vi "main_ctrl.vi"(8 "error in":errorcluster) -> (0 "error out":errorcluster caption="error")   [LabVIEW 2013]
uses:
  <vilib>/Rock Robotics/WPI/DriverStation/WPI_DriverStationRobotMode.ctl
  typedefs/fg_typedef.ctl
  typedefs/vision enable.ctl
  typedefs/subStates.ctl
  typedefs/singleUseSubstate.ctl
  <vilib>/Rock Robotics/WPI/Solenoid/WPI_SolenoidValue.ctl
  <vilib>/Rock Robotics/WPI/Compressor/WPI_CompressorGetSetRefNum.vi
  <vilib>/Rock Robotics/WPI/RobotDrive/WPI_RobotDriveGetSetRefNum.vi
  <vilib>/Rock Robotics/WPI/RobotDrive/WPI_RobotDriveArcadeDrive_Standard(NoSaturation).vi
  <vilib>/Rock Robotics/WPI/Solenoid/WPI_SolenoidSetEnum.vi
panel:
  out "Robot Mode":T1
  out "Vision SPI":u32
  out "Vision IPS":dbl
  out "Main IPS":dbl
  out "Main SPI":u32
  # "MAIN CONTROL"
  # "holds robot control code - dual parallel state machine"
  # "SPI: milliseconds per iteration\nIPS: iterations per second"
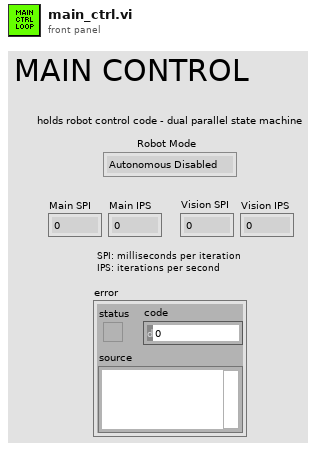
[diagram p1: front panel]
types:
  T1 = typedef "WPI_DriverStationRobotMode.ctl" = enum16{"Autonomous Disabled", "Autonomous Enabled", "Teleop Disabled", "Teleop Enabled", "Timeout", "Finish"}
  T2 = typedef "WPI_RobotDriveDevRef.ctl" = cluster{"DevStatus":errorcluster, "Motors[]":T3[], "Square Inputs":bool, "Max Output":dbl, "Isochronous":bool}
  T3 = typedef "WPI_MotorControlDeviceRef.ctl" = cluster{"DeviceStatus":errorcluster, "Type":enum16{"PWM", "CAN"}, "PWM":cluster{"Digital Module":T4, "PWM Channel":T5, "DeadBand":T6}, "CAN":cluster{"Device Number":u8, "Control Mode":T7, "Semaphore":T8, "Max Vout":dbl}, "Invert":bool, "TransformRef":T9, "InvTransformRef":T9}
  T4 = typedef "FPGA_TypedefDigitalModule.ctl" = enum16{"Digital Module 1", "Digital Module 2"}
  T5 = typedef "FPGA_DIOPWMChannel.ctl" = enum8{"PWM 1", "PWM 2", "PWM 3", "PWM 4", "PWM 5", "PWM 6", "PWM 7", "PWM 8", "PWM 9", "PWM 10", "Invalid"}
  T6 = typedef "WPI_PWMDeadband.ctl" = cluster{"Name":string, "maxPositivePwm":i32, "minPositivePwm":i32, "centerPwm":i32, "maxNegativePwm":i32, "minNegativePwm":i32, "angularRange":u16}
  T7 = typedef "WPI_CANJaguar_ControlMode.ctl" = enum8{"Percent VBus", "Current", "Speed", "Position", "Voltage"}
  T8 = typedef "Semaphore RefNum" = refnum<k1>
  T9 = typedef "WPI_PWMTransform_ConPane.ctl" = refnum<vi>
  T10 = typedef "WPI_CompressorDevRef.ctl" = cluster{"DevStatus":errorcluster, "DigitalInputDevRef":T11, "RelayDevRef":T13}
  T11 = typedef "WPI_DigitalInputDevRef.ctl" = cluster{"DevStatus":errorcluster, "DIO Channel":T12, "Digital Module":T4}
  T12 = typedef "FPGA_DIOChannel.ctl" = enum8{"DIO 1", "DIO 2", "DIO 3", "DIO 4", "DIO 5", "DIO 6", "DIO 7", "DIO 8", "DIO 9", "DIO 10", "DIO 11", "DIO 12", "DIO 13", "DIO 14", "Invalid"}
  T13 = typedef "WPI_RelayDevRef.ctl" = cluster{"DevStatus":errorcluster, "Relay Channel":T14, "Digital Module":T4, "Relay Direction":T15}
  T14 = typedef "FPGA_DIORelayChannel.ctl" = enum8{"Relay 1", "Relay 2", "Relay 3", "Relay 4", "Relay 5", "Relay 6", "Relay 7", "Relay 8", "Invalid"}
  T15 = typedef "WPI_RelayDirection.ctl" = enum16{"Both directions", "Forward only", "Reverse only"}
  T16 = cluster{"Left":dbl, "Top":dbl, "Right":dbl, "Bottom":dbl, "Target CoM X":dbl, "Target CoM Y":dbl}
  T17 = typedef "vision enable.ctl" = enum16{"Enable", "Disable", "Stop"}
  T18 = typedef "fg_typedef.ctl" = enum16{"Get", "Set"}
  T19 = typedef "WPI_CameraDevRef.ctl" = cluster{"Camera Address":string, "CameraStatus":errorcluster, "Acquire Image Notifier":refnum<notifier>}
  T20 = typedef "IMAQ Image.ctl" = refnum<image>
  T21 = cluster{"Vision mSPI":u32, "Main mSPI":u32, "Dash mSPI":u32}
  T22 = typedef "WPI_SolenoidDevRef.ctl" = cluster{"DevStatus":errorcluster, "Solenoid Module":T23, "Forward Solenoid Channel":T24, "Reverse Solenoid Channel":T24}
  T23 = typedef "FPGA_TypedefSolenoidModule.ctl" = enum16{"Solenoid Module 1", "Solenoid Module 2"}
  T24 = typedef "WPI_SolenoidChannel.ctl" = enum8{"Solenoid 1", "Solenoid 2", "Solenoid 3", "Solenoid 4", "Solenoid 5", "Solenoid 6", "Solenoid 7", "Solenoid 8", "Invalid"}
  T25 = typedef "WPI_SolenoidValue.ctl" = enum16{"Off", "On", "Forward", "Reverse"}
  T26 = typedef "singleUseSubstate.ctl" = enum16{"null", "wait", "shift high", "shift low"}
  T27 = typedef "WPI_DriverStationDerivedRobotMode.ctl" = enum16{"Init", "Execute", "Stop"}
  T28 = typedef "subStates.ctl" = enum16{"null", "wait", "driver control", "auto", "manual override", "hold position", "rotate", "feeder", "shoot", "end"}
  T29 = typedef "Loop 2 Datatype.ctl" = cluster{"State":T28, "Waiting Loop":i32, "State to Wait For":i32, "Loop ID":i32, "Exit Value":i32, "Joystick":dbl}
  T30 = typedef "Loop 1 Datatype.ctl" = cluster{"State":T28, "Waiting Loop":i32, "State to Wait For":i32, "Loop ID":i32, "Exit Value":i32, "Joystick":dbl, "Index Up":bool, "Index Down":bool}
  T31 = typedef "Loop 3 Datatype.ctl" = cluster{"State":T28, "Waiting Loop":i32, "State to Wait For":i32, "Loop ID":i32, "Exit Value":i32, "Joystick":dbl, "Z Axis":dbl}
  T32 = typedef "Loop 0 Datatype.ctl" = cluster{"State":T28, "Waiting Loop":i32, "State to Wait For":i32, "Loop ID":i32, "Exit Value":i32, "X Axis":dbl, "Y Axis":dbl, "Z Axis":dbl}
  T33 = typedef "Loop 4 Datatype.ctl" = cluster{"State":T28, "Waiting Loop":i32, "State to Wait For":i32, "Loop ID":i32, "Exit Value":i32, "Joystick":dbl}
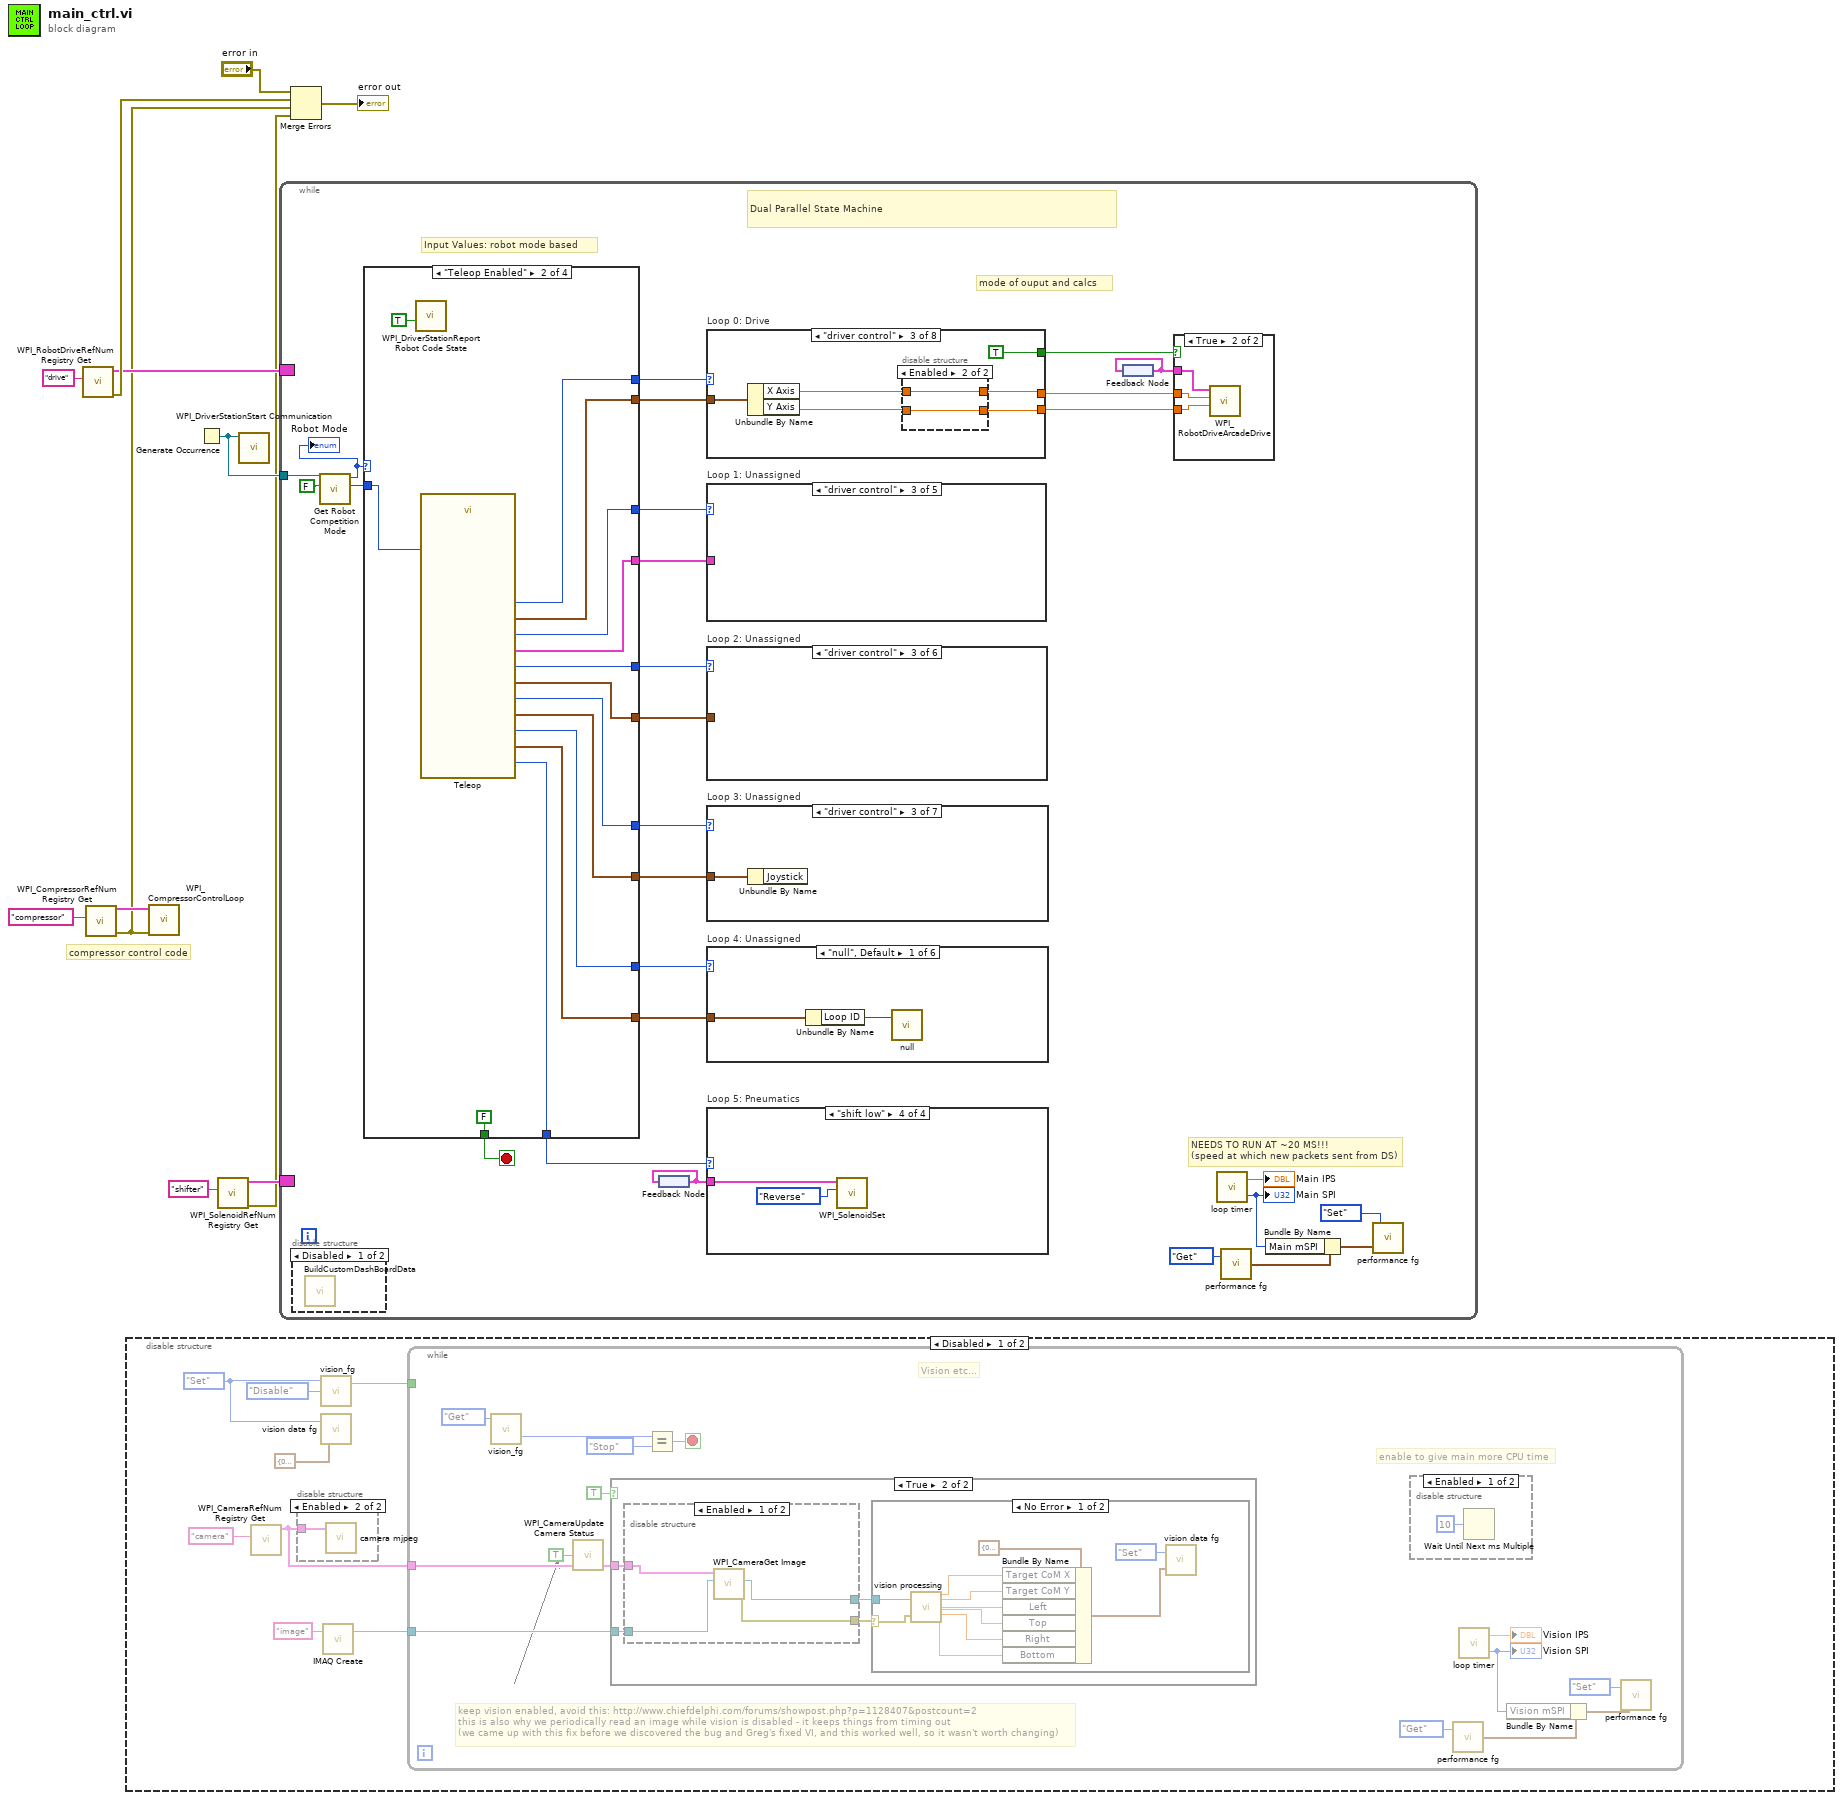
[diagram p0: block diagram]
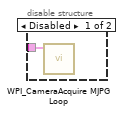
[diagram p2: hidden frame]
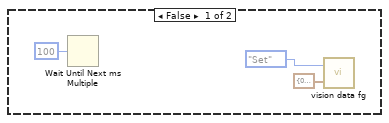
[diagram p4: hidden frame]
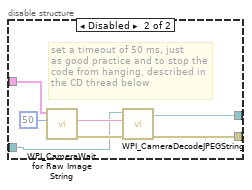
[diagram p6: hidden frame]
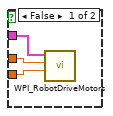
[diagram p9: hidden frame]
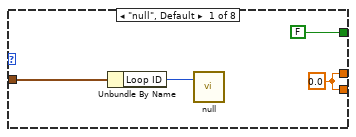
[diagram p10: hidden frame]
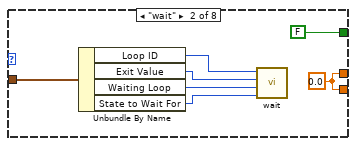
[diagram p11: hidden frame]
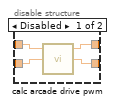
[diagram p12: hidden frame]
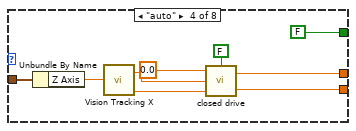
[diagram p13: hidden frame]
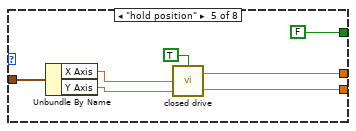
[diagram p14: hidden frame]
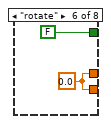
[diagram p15: hidden frame]
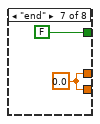
[diagram p16: hidden frame]
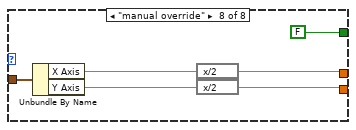
[diagram p17: hidden frame]
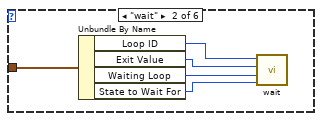
[diagram p18: hidden frame]
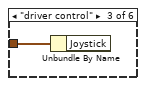
[diagram p19: hidden frame]
diagram:
  # "compressor control code"
  n1 = call <vilib>:"WPI_RobotDriveRefNum Registry Get.vi"("refnum name"="drive") -> ("error out"=w8:errorcluster, "RobotDriveDevRef"=w6:T2)  [unwired: 9 in]
  n2 = call <vilib>:"WPI_CompressorRefNum Registry Get.vi"("refnum name"="compressor") -> ("error out"=w2:errorcluster, "CompressorDevRef"=w5:T10)  [unwired: 9 in]
  n3 = disable-structure shown="Disabled" {
    frame Disabled {
      w18 = fg_typedef."Set" ("Enum")
      n4 = call <vilib>:"WPI_CameraRefNum Registry Get.vi"("refnum name"="camera") -> ("CameraDevRef"=w15:T19)  [unwired: 9 in, 1 out]
      n5 = disable-structure shown="Enabled" {
        disable-tunnel: w15 -> [w21 w22]
        frame Disabled {
          n6 = call <vilib>:"WPI_CameraAcquire MJPG Loop.vi"("CameraDevRef"=w21) -> ()  [unwired: 11 in]
        }
        frame Enabled {
          n7 = call "camera mjpeg.vi"("CameraDevRef"=w22) -> ()  [unwired: 11 in]
        }
      }
      n8 = call "vision_fg.vi"("Action"=vision_enable."Disable", "Menu"=w18) -> ("Enabled?"=w19:bool)  [unwired: 1 in, 1 out]
      n9 = call "vision data fg.vi"("Input"=T16 {"Left"=0.0, "Top"=0.0, "Right"=0.0, "Bottom"=0.0, "Target CoM X"=0.0, "Target CoM Y"=0.0}, "Menu"=w18) -> ()  [unwired: 1 out]
      n10 = call "IMAQ Create"("Image Name"="image") -> ("New Image"=w20:T20)  [unwired: 4 in, 1 out]
      n11 = while {
        tunnel: w20 -> [w36]
        tunnel: w15 -> [w35]
        tunnel: w19 -> [_]
        stop <- w37 stop-if-true
        # "keep vision enabled, avoid this: http://www.chiefdelphi.com/forums/showpost.php?p=1128407&postcount=2\nthis is also why we periodically read an image while vision is disabled - it keeps things from timing out\n(we came up with this fix before we discovered the bug and Greg's fixed VI, and this worked well, so it wasn't worth changing)"
        # "enable to give main more CPU time"
        # "Vision etc..."
        n12 = call "vision_fg.vi"("Menu"=fg_typedef."Get" ("Enum")) -> ("State Out"=w31:T17)  [unwired: 2 in, 1 out]
        n13 = call <vilib>:"WPI_CameraUpdate Camera Status.vi"("CameraDevRef In"=w35, "Enable Vision"=TRUE) -> ("CameraDevRef Out"=w34:T19)  [unwired: 3 in]
        n14 = case shown="True" TRUE {
          tunnel: w36 -> [_ w45]
          tunnel: w34 -> [_ w44]
          frame False {
            n15 = Wait Until Next ms Multiple(millisecond multiple=u32 100) -> ()  [unwired: 1 out]
            n16 = call "vision data fg.vi"("Input"=T16 {"Left"=0.0, "Top"=0.0, "Right"=0.0, "Bottom"=0.0, "Target CoM X"=0.0, "Target CoM Y"=0.0}, "Menu"=fg_typedef."Set" ("Enum")) -> ()  [unwired: 1 out]
          }
          frame True {
            n17 = disable-structure shown="Enabled" {
              disable-tunnel: w45 -> [w59 w63]
              disable-tunnel: w44 -> [w60 w65]
              disable-tunnel: [w58 w62] -> w43
              disable-tunnel: [w57 w61] -> w42
              frame Enabled {
                n18 = call <vilib>:"WPI_CameraGet Image.vi"("Image"=w59, "CameraDevRef"=w60) -> ("error out"=w57:errorcluster, "Image Out"=w58:T20)  [unwired: 7 in, 1 out]
              }
              frame Disabled {
                # "set a timeout of 50 ms, just\nas good practice and to stop the \ncode from hanging, described in \nthe CD thread below"
                n19 = call <vilib>:"WPI_CameraWait for Raw Image String.vi"("Timeout in ms (-1)"=50, "CameraDevRef"=w65) -> ("error out"=w67:errorcluster, "String"=w66:string)  [unwired: 3 in, 5 out]
                n20 = call <vilib>:"WPI_CameraDecodeJPEGString.vi"("error in"=w67, "Compressed Image"=w66, "Image In"=w63) -> ("error out"=w61:errorcluster, "Image Out"=w62:T20)  [unwired: 3 out]
              }
            }
            n21 = case shown="No Error" w42 {
              selector: w42 -> [w54 _]
              tunnel: w43 -> [w55 _]
              frame No Error {
                n22 = call "vision processing.vi"("Image In"=w55, "error in (no error)"=w54) -> ("x"=w53:dbl, "y"=w52:dbl, "left"=w50:dbl, "top"=w49:dbl, "right"=w48:dbl, "bottom"=w47:dbl)  [unwired: 11 in, 1 out]
                n23 = Bundle By Name(cluster=T16 {"Left"=0.0, "Top"=0.0, "Right"=0.0, "Bottom"=0.0, "Target CoM X"=0.0, "Target CoM Y"=0.0} ("Input"), "Target CoM X"=w53, "Target CoM Y"=w52, "Left"=w50, "Top"=w49, "Right"=w48, "Bottom"=w47) -> (w46:T16)
                n24 = call "vision data fg.vi"("Input"=w46, "Menu"=fg_typedef."Set" ("Enum")) -> ()  [unwired: 1 out]
              }
              frame Error {
              }
            }
          }
        }
        n25 = Equal?(x=w31, y=vision_enable."Stop") -> (x = y?=w37:bool)
        n26 = disable-structure shown="Enabled" {
          frame Enabled {
            n27 = Wait Until Next ms Multiple(millisecond multiple=u32 10) -> ()  [unwired: 1 out]
          }
          frame Disabled {
          }
        }
        n28 = call "performance fg.vi"("Menu"=fg_typedef."Get") -> ("Output"=w27:T21)  [unwired: 1 in]
        n29 = call "loop timer.vi"() -> ("IPS"=→"Vision IPS":dbl, "SPI"=w29:u32)  [unwired: 1 in]
        "Vision SPI" <- w29
        n30 = Bundle By Name(cluster=w27, "Vision mSPI"=w29) -> (w26:T21)
        n31 = call "performance fg.vi"("Input"=w26, "Menu"=fg_typedef."Set") -> ()  [unwired: 1 out]
      }
    }
    frame Enabled {
    }
  }
  n32 = call <vilib>:"WPI_CompressorControlLoop.vi"("error in (no error)"=w2, "CompressorDevRef"=w5) -> ()  [unwired: 10 in]
  n33 = Generate Occurrence() -> (w12:refnum<k4>)
  n34 = call <vilib>:"WPI_SolenoidRefNum Registry Get.vi"("refnum name"="shifter") -> ("error out"=w1:errorcluster, "SolenoidDevRef"=w4:T22)  [unwired: 9 in]
  n35 = call <vilib>:"WPI_DriverStationStart Communication.vi"("occurrence"=w12) -> ()  [unwired: 11 out]
  n36 = while {
    tunnel: w12 -> [w93]
    border: w6 -> [_]
    border: w4 -> [_]
    stop <- w87 stop-if-true
    # "Input Values: robot mode based"
    # "mode of ouput and calcs"
    # "NEEDS TO RUN AT ~20 MS!!!\n(speed at which new packets sent from DS)"
    # "Dual Parallel State Machine"
    n37 = disable-structure shown="Disabled" {
      frame Disabled {
        n38 = call "BuildCustomDashBoardData.vi"() -> ()  [unwired: 12 in]
      }
      frame Enabled {
      }
    }
    n39 = call "Get Robot Competition Mode.vi"("Finish"=FALSE, "DS Occurrence"=w93) -> ("Call Context"=w91:T27, "Robot Mode"=w92:T1)  [unwired: 6 in, 2 out]
    "Robot Mode" <- w92
    n40 = case shown="\"Teleop Enabled\"" w92 {
      tunnel: [w199 w217 w218 w224] -> w68
      tunnel: w91 -> [w190 w212 _ _]
      tunnel: [w197 w216 w218 w224] -> w89
      tunnel: [w191 w214 singleUseSubstate."null" ("SubState 5") singleUseSubstate."null" ("SubState 5")] -> w88
      tunnel: [FALSE FALSE FALSE TRUE] -> w87
      tunnel: [w201 w211 w218 w224] -> w80
      tunnel: [w200 w210 _ _] -> w81
      tunnel: [w198 w209 _ _] -> w79
      tunnel: [w196 w208 _ _] -> w78
      tunnel: [w194 w207 _ _] -> w76
      tunnel: [w192 w206 _ _] -> w75
      tunnel: [w193 w205 w218 w224] -> w74
      tunnel: [w195 w204 w218 w224] -> w73
      frame "Autonomous Enabled" {
        n41 = call <vilib>:"WPI_DriverStationReport Robot Code State.vi"("Autonomous"=TRUE) -> ()  [unwired: 10 in, 1 out]
        n42 = call "Autonomous.vi"("Call Context"=w190) -> ("SubState 2"=w197:T28, "Loop 2 Data"=w196:T29, "SubState 1"=w199:T28, "Loop 1 Data"=w198:T30, "Loop 3 Data"=w194:T31, "SubState 0"=w201:T28, "SubState 3"=w195:T28, "Loop 0 Data"=w200:T32, "Loop 4 Data"=w192:T33, "SubState 4"=w193:T28, "SubState 5"=w191:T26)
      }
      frame "Teleop Enabled" {
        n43 = call <vilib>:"WPI_DriverStationReport Robot Code State.vi"("TeleOp"=TRUE) -> ()  [unwired: 10 in, 1 out]
        n44 = call "Teleop.vi"("Call Context"=w212) -> ("SubState 3"=w204:T28, "SubState 4"=w205:T28, "SubState 5"=w214:T26, "Loop 3 Data"=w207:T31, "Loop 4 Data"=w206:T33, "SubState 0"=w211:T28, "Loop 1 Data"=w209:T30, "Loop 0 Data"=w210:T32, "SubState 1"=w217:T28, "Loop 2 Data"=w208:T29, "SubState 2"=w216:T28)  [unwired: 8 in]
      }
      frame "Autonomous Disabled", "Teleop Disabled", "Timeout" {
        w218 = subStates."null" ("SubState 0")
        # "set all loops to null"
        # "make sure to disable vision\nwe don't need it here"
        # "robot disabled, timeout"
        n45 = call <vilib>:"WPI_DriverStationReport Robot Code State.vi"("Disabled"=TRUE) -> ()  [unwired: 10 in, 1 out]
        n46 = call "vision_fg.vi"("Action"=vision_enable."Disable", "Menu"=fg_typedef."Set") -> ()  [unwired: 1 in, 2 out]
      }
      frame "Finish" {
        w224 = subStates."end"  # Stop All Loops
        # "stop the while loop"
        # "stop DS comms"
        # "stop vision loop"
        n47 = call <vilib>:"WPI_DriverStationStop Communication.vi"("StopCommunication"=TRUE) -> ()  [unwired: 10 in, 1 out]
        n48 = call "vision_fg.vi"("Action"=vision_enable."Stop", "Menu"=fg_typedef."Set") -> ()  [unwired: 1 in, 2 out]
      }
    }
    n49 = feedback #1() -> (w77:T22)
    n50 = feedback-in #1(w77) -> ()
    n51 = case "Loop 0: Drive" shown="\"driver control\"" w80 {
      tunnel: w81 -> [w103 w107 w117 w126 w138 _ _ w149]
      tunnel: [w101 w105 w113 w131 w135 w141 w143 w145] -> w71
      tunnel: [w101 w105 w112 w130 w134 w141 w143 w144] -> w70
      tunnel: [FALSE FALSE TRUE FALSE FALSE FALSE FALSE FALSE] -> w72
      frame "null", Default {
        w101 = 0.0 ("X Axis")
        n52 = Unbundle By Name(w103) -> ("Loop ID"=w104:i32)
        n53 = call "null.vi"("This Loop ID"=w104) -> ()  [unwired: 2 in]
      }
      frame "wait" {
        w105 = 0.0 ("X Axis")
        n54 = Unbundle By Name(w107) -> ("Loop ID"=w111:i32, "Exit Value"=w110:i32, "Waiting Loop"=w109:i32, "State to Wait For"=w108:i32)
        n55 = call "wait.vi"("State to wait for"=w108, "Waiting Loop ID"=w109, "time (ms)"=w110, "Current Loop ID"=w111) -> ()  [unwired: 1 out]
      }
      frame "driver control" {
        n56 = Unbundle By Name(w117) -> ("X Axis"=w115:dbl, "Y Axis"=w114:dbl)
        n57 = disable-structure shown="Enabled" {
          disable-tunnel: w115 -> [w121 w123]
          disable-tunnel: w114 -> [w120 w122]
          disable-tunnel: [w119 w123] -> w113
          disable-tunnel: [w118 w122] -> w112
          frame Disabled {
            n58 = call "calc arcade drive pwm.vi"("Y axis value"=w120, "X axis value"=w121) -> ("Right Speed"=w118:dbl, "Left Speed"=w119:dbl)  [unwired: 1 in, 1 out]
          }
          frame Enabled {
          }
        }
      }
      frame "auto" {
        n59 = Unbundle By Name(w126) -> ("Z Axis"=w125:dbl)
        n60 = call "Vision Tracking X.vi"("Tweak"=w125) -> ("right speed"=w124:dbl, "left speed"=w128:dbl)
        n61 = call "closed drive.vi"("Acrade Drive?"=FALSE, "Y axis value (Left)"=w128, "X axis value (Right)"=w124, "Threshold (.4)"=0.0 ("Threshold")) -> ("right"=w130:dbl, "left"=w131:dbl)
      }
      frame "hold position" {
        n62 = Unbundle By Name(w138) -> ("X Axis"=w137:dbl, "Y Axis"=w136:dbl)
        n63 = call "closed drive.vi"("Acrade Drive?"=TRUE, "Y axis value (Left)"=w136, "X axis value (Right)"=w137) -> ("right"=w134:dbl, "left"=w135:dbl)  [unwired: 1 in]
      }
      frame "rotate" {
        w141 = 0.0 ("X Axis")
      }
      frame "end" {
        w143 = 0.0 ("X Axis")
      }
      frame "manual override" {
        n64 = Unbundle By Name(w149) -> ("X Axis"=w148:dbl, "Y Axis"=w147:dbl)
        n65 = expression code="x/2"(w148) -> (w145:dbl)
        n66 = expression code="x/2"(w147) -> (w144:dbl)
      }
    }
    n67 = case "Loop 1: Unassigned" shown="\"driver control\"" w68 {
      tunnel: w79 -> [w182 w184 _ _ w189]
      frame "null", Default {
        n68 = Unbundle By Name(w182) -> ("Loop ID"=w183:i32)
        n69 = call "null.vi"("This Loop ID"=w183) -> ()  [unwired: 2 in]
      }
      frame "wait" {
        n70 = Unbundle By Name(w184) -> ("Loop ID"=w188:i32, "Exit Value"=w187:i32, "Waiting Loop"=w186:i32, "State to Wait For"=w185:i32)
        n71 = call "wait.vi"("State to wait for"=w185, "Waiting Loop ID"=w186, "time (ms)"=w187, "Current Loop ID"=w188) -> ()  [unwired: 1 out]
      }
      frame "driver control" {
      }
      frame "auto" {
      }
      frame "manual override" {
        n72 = Unbundle By Name(w189) -> ()  [unwired: 1 out]
      }
    }
    n73 = case "Loop 2: Unassigned" shown="\"driver control\"" w89 {
      tunnel: w78 -> [w175 w176 _ _ w181 _]
      frame "null", Default {
        n74 = Unbundle By Name(w175) -> ("Loop ID"=w174:i32)
        n75 = call "null.vi"("This Loop ID"=w174) -> ()  [unwired: 2 in]
      }
      frame "wait" {
        n76 = Unbundle By Name(w176) -> ("Loop ID"=w180:i32, "Exit Value"=w179:i32, "Waiting Loop"=w178:i32, "State to Wait For"=w177:i32)
        n77 = call "wait.vi"("State to wait for"=w177, "Waiting Loop ID"=w178, "time (ms)"=w179, "Current Loop ID"=w180) -> ()  [unwired: 1 out]
      }
      frame "driver control" {
      }
      frame "auto" {
      }
      frame "manual override" {
        n78 = Unbundle By Name(w181) -> ()  [unwired: 1 out]
      }
      frame "feeder" {
      }
    }
    n79 = case "Loop 3: Unassigned" shown="\"driver control\"" w73 {
      tunnel: w76 -> [w160 w161 w166 _ w167 w168 w169]
      frame "null", Default {
        n80 = Unbundle By Name(w160) -> ("Loop ID"=w159:i32)
        n81 = call "null.vi"("This Loop ID"=w159) -> ()  [unwired: 2 in]
      }
      frame "wait" {
        n82 = Unbundle By Name(w161) -> ("Loop ID"=w165:i32, "Exit Value"=w164:i32, "Waiting Loop"=w163:i32, "State to Wait For"=w162:i32)
        n83 = call "wait.vi"("State to wait for"=w162, "Waiting Loop ID"=w163, "time (ms)"=w164, "Current Loop ID"=w165) -> ()  [unwired: 1 out]
      }
      frame "driver control" {
        n84 = Unbundle By Name(w166) -> ()  [unwired: 1 out]
      }
      frame "auto" {
      }
      frame "manual override" {
        n85 = Unbundle By Name(w167) -> ()  [unwired: 1 out]
      }
      frame "feeder" {
        n86 = Unbundle By Name(w168) -> ()  [unwired: 1 out]
      }
      frame "shoot" {
        n87 = Unbundle By Name(w169) -> ()  [unwired: 1 out]
      }
    }
    n88 = case "Loop 4: Unassigned" shown="\"null\", Default" w74 {
      tunnel: w75 -> [w151 w152 w157 _ w158 _]
      frame "null", Default {
        n89 = Unbundle By Name(w151) -> ("Loop ID"=w150:i32)
        n90 = call "null.vi"("This Loop ID"=w150) -> ()  [unwired: 2 in]
      }
      frame "wait" {
        n91 = Unbundle By Name(w152) -> ("Loop ID"=w156:i32, "Exit Value"=w155:i32, "Waiting Loop"=w154:i32, "State to Wait For"=w153:i32)
        n92 = call "wait.vi"("State to wait for"=w153, "Waiting Loop ID"=w154, "time (ms)"=w155, "Current Loop ID"=w156) -> ()  [unwired: 1 out]
      }
      frame "driver control" {
        n93 = Unbundle By Name(w157) -> ()  [unwired: 1 out]
      }
      frame "auto" {
      }
      frame "manual override" {
        n94 = Unbundle By Name(w158) -> ()  [unwired: 1 out]
      }
      frame "feeder" {
      }
    }
    n95 = case "Loop 5: Pneumatics" shown="\"shift low\"" w88 {
      tunnel: w77 -> [_ _ w171 w172]
      frame "null", Default {
      }
      frame "wait" {
      }
      frame "shift high" {
        n96 = call-poly <vilib>:"WPI_SolenoidSet.vi"("Value"=WPI_SolenoidValue."Forward", "SolenoidDevRef"=w171) -> ()  [unwired: 8 in, 2 out]
      }
      frame "shift low" {
        n97 = call-poly <vilib>:"WPI_SolenoidSet.vi"("Value"=WPI_SolenoidValue."Reverse", "SolenoidDevRef"=w172) -> ()  [unwired: 8 in, 2 out]
      }
    }
    n98 = feedback #2() -> (w69:T2)
    n99 = feedback-in #2(w69) -> ()
    n100 = case shown="True" w72 {
      tunnel: w71 -> [w96 w100]
      tunnel: w70 -> [w95 w99]
      tunnel: w69 -> [w97 w98]
      frame False {
        n101 = call <vilib>:"WPI_RobotDriveMotors.vi"("RightSpeed"=w95, "LeftSpeed"=w96, "RobotDriveDevRef"=w97) -> ()  [unwired: 6 in, 3 out]
      }
      frame True {
        n102 = call-poly <vilib>:"WPI_RobotDriveArcadeDrive.vi"("Y axis value"=w99, "X axis value"=w100, "RobotDriveDevRef"=w98) -> ()  [unwired: 6 in, 3 out]
      }
    }
    n103 = call "loop timer.vi"() -> ("IPS"=→"Main IPS":dbl, "SPI"=w86:u32)  [unwired: 1 in]
    "Main SPI" <- w86
    n104 = call "performance fg.vi"("Menu"=fg_typedef."Get") -> ("Output"=w83:T21)  [unwired: 1 in]
    n105 = Bundle By Name(cluster=w83, "Main mSPI"=w86) -> (w82:T21)
    n106 = call "performance fg.vi"("Input"=w82, "Menu"=fg_typedef."Set") -> ()  [unwired: 1 out]
  }
  n107 = Merge Errors("error in", w8, w2, w1) -> (→"error out":errorcluster)
